vi "Open DAQ File.vi"(3 "EXE distribution?":bool=TRUE, 5 "start path":path) -> (0 "error out":errorcluster, 1 "new file path":path, 2 "refnum out":refnum<file>)   [LabVIEW 2017]
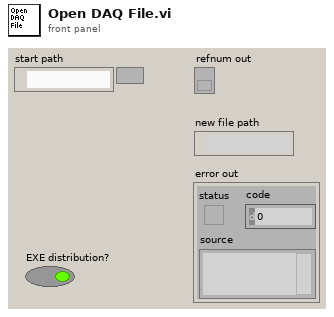
[diagram p1: front panel]
types:
  T1 = enum16{"open", "open or create", "create or replace", "create", "open (read only)"}
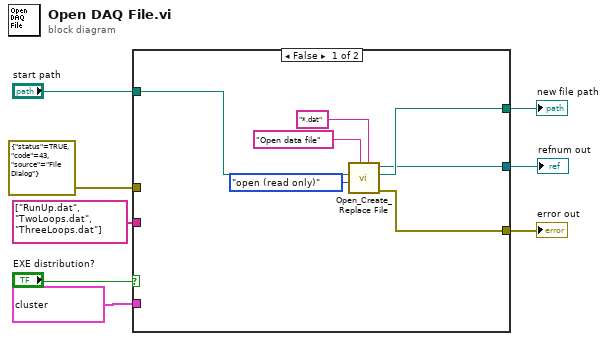
[diagram p0: block diagram]
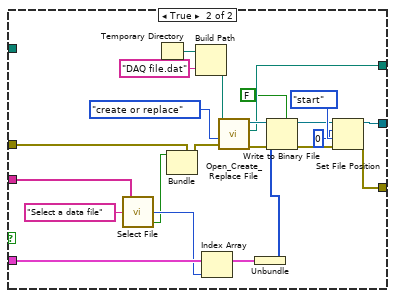
[diagram p2: hidden frame]
diagram:
  n1 = case shown="False" "EXE distribution?" {
    tunnel: [w15 w32] -> w8
    tunnel: "start path" -> [w14 _]
    tunnel: [w13 w28] -> w6
    tunnel: [w12 w25] -> w5
    tunnel: cluster{u8[]}[] [{array[387169 elements]}, {array[647291 elements]}, {array[589947 elements]}] ("DAQ Data") -> [_ w37]
    tunnel: errorcluster {"status"=TRUE, "code"=43, "source"="File Dialog"} ("error out") -> [_ w30]
    tunnel: string[] ["RunUp.dat", "TwoLoops.dat", "ThreeLoops.dat"] ("Item Names") -> [_ w18]
    frame False {
      n2 = call <vilib>:"Open_Create_Replace File.vi"("pattern"="*.dat", "prompt"="Open data file", "function (open:0)"=T1."open (read only)", "start path  (Not A Path)"=w14) -> ("error out"=w12:errorcluster, "new file path"=w15:path, "refnum"=w13:refnum<file>)  [unwired: 4 in, 1 out]
    }
    frame True {
      n3 = call <vilib>:"Select File.vi"("prompt"="Select a data file", "file names"=w18) -> ("canceled"=w19:bool, "index"=w20:i32)  [unwired: 1 in, 1 out]
      n4 = Temporary Directory() -> (w35:path)
      n5 = Bundle(cluster=w30, "status"=w19) -> (w29:errorcluster)  [unwired: 2 in]
      n6 = Build Path(base path=w35, name or relative path="DAQ file.dat") -> (appended path=w33:path)
      n7 = Index Array(array=w37, index=w20) -> (element=w24:cluster{u8[]})
      n8 = call <vilib>:"Open_Create_Replace File.vi"("error in (no error)"=w29, "function (open:0)"=T1."create or replace", "file path"=w33) -> ("error out"=w36:errorcluster, "new file path"=w32:path, "refnum"=w38:refnum<file>)  [unwired: 5 in, 1 out]
      n9 = Unbundle(w24) -> (w23:u8[])
      n10 = Write to Binary File(file (use dialog)=w38, data=w23, error in=w36, 5:FALSE ("prepend array or string size? (T)")) -> (refnum out=w22:refnum<file>, error out=w21:errorcluster)  [unwired: 2 in, 1 out]
      n11 = Set File Position(offset (in bytes) (0)=0 ("pos offset (0)"), refnum=w22, from (0:start)=enum16{"start", "end", "current"}."start" ("pos mode (0:2)"), error in=w21) -> (refnum out=w28:refnum<file>, error out=w25:errorcluster)
    }
  }
  "new file path" <- w8
  "refnum out" <- w6
  "error out" <- w5
